vi "Connect.vi"(8 "error in (no error)":errorcluster, 11 "ImageHandler in":refnum<class "ImageHandler.lvclass">) -> (0 "error out":errorcluster, 1 "Serial Number":string, 2 "Sensor Status":i32, 3 "ImageHandler out":refnum<class "ImageHandler.lvclass">)   [LabVIEW 2022 SP3, in "ImageHandler.lvlib" / "ImageHandler.lvclass"]
uses:
  ImageHandler.lvclass
  C:/Program Files/National Instruments/LabVIEW 2022/vi.lib/ActorFramework/Actor/Actor.lvclass
  <vilib>/ActorFramework/Actor/Actor.lvclass/Actor.ctl
  ImageHandler.lvclass/ImageHandler.ctl
  ImageHandler - Controller -- Interface/ImageHandler - Controller -- Interface Messages/Log Message Msg/Log Message Msg.lvclass/Log Message Msg.ctl
  <vilib>/ActorFramework/Message Enqueuer/Message Enqueuer.lvclass/Message Enqueuer.ctl
  <vilib>/ActorFramework/Message Enqueuer/Enqueue.vi
  ImageHandler - Controller -- Interface/ImageHandler - Controller -- Interface Messages/Log Message Msg/Log Message Msg.lvclass
  C:/Program Files/National Instruments/LabVIEW 2022/vi.lib/ActorFramework/Message/Message.lvclass
  <vilib>/ActorFramework/Message Priority Queue/Priority Enqueue.vi
  BonTechDetector/BonTechDetector.lvlib
  <vilib>/ActorFramework/Actor/Actor.lvclass
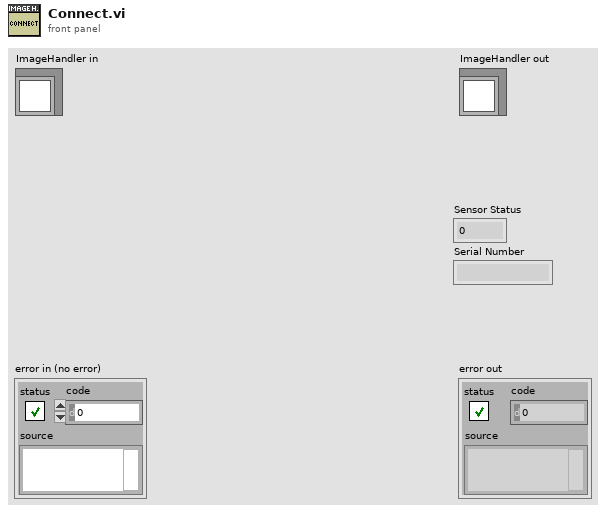
[diagram p1: front panel]
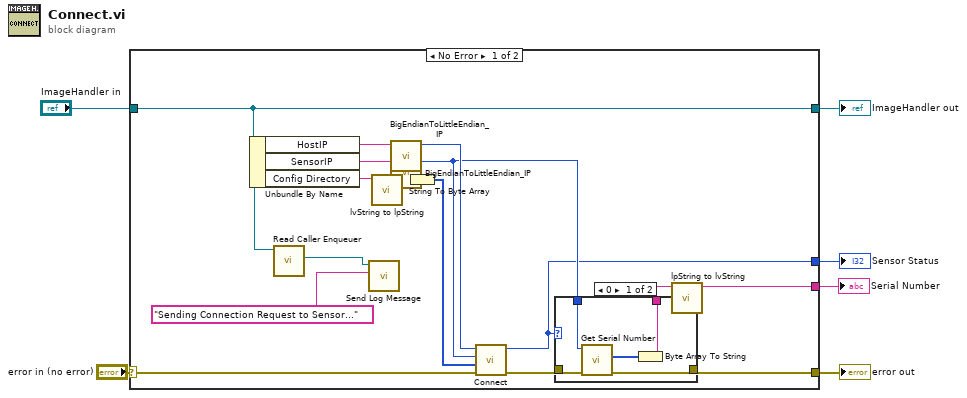
[diagram p0: block diagram]
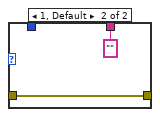
[diagram p2: hidden frame]
diagram:
  n1 = case shown="No Error" "error in (no error)" {
    selector: "error in (no error)" -> [w20 w31]
    tunnel: [w12 w31] -> w5
    tunnel: [w9 w30] -> w3
    tunnel: "ImageHandler in" -> [w9 w30]
    tunnel: [w10 _] -> w2
    tunnel: [w11 _] -> w1
    frame No Error {
      n2 = Unbundle By Name(w9) -> ("HostIP"=w22:string, "SensorIP"=w19:string, "Config Directory"=w18:string)
      n3 = call <vilib>:"Read Caller Enqueuer.vi"("Actor"=w9) -> ("Caller Enqueuer"=w8:refnum<class "Message Enqueuer.lvclass">)  [unwired: 10 in]
      n4 = call "Send Log Message.vi"("Log Message"="Sending Connection Request to Sensor...", "Message Enqueuer"=w8) -> ()  [unwired: 8 in, 2 out]
      n5 = call "lvString to lpString.vi"("LVString"=w18) -> ("LPTSTR String"=w17:string)  [unwired: 10 in]
      n6 = call "BigEndianToLittleEndian_IP.vi"("IP String"=w22) -> ("IP Network Order"=w21:u32)  [unwired: 10 in]
      n7 = call "BigEndianToLittleEndian_IP.vi"("IP String"=w19) -> ("IP Network Order"=w14:u32)  [unwired: 10 in]
      n8 = String To Byte Array(string=w17) -> (unsigned byte array=w16:u8[])
      n9 = call "Connect.vi"("error in (no error)"=w20, "ConfigDir"=w16, "nSensorIP"=w14, "nHostIP"=w21) -> ("error out"=w13:errorcluster, "function return"=w10:i32)  [unwired: 6 in]
      n10 = case shown="0" w10 {
        tunnel: [w27 "" ("string")] -> w15
        tunnel: w14 -> [w25 _]
        tunnel: w13 -> [w24 w29]
        tunnel: [w23 w29] -> w12
        frame 0 {
          n11 = call "Get Serial Number.vi"("error in (no error)"=w24, "nSensorIP"=w25) -> ("error out"=w23:errorcluster, "lpszSerialNum out"=w26:u8[])  [unwired: 7 in, 1 out]
          n12 = Byte Array To String(unsigned byte array=w26) -> (string=w27:string)
        }
        frame 1, Default {
        }
      }
      n13 = call "lpString to lvString.vi"("LPTSTR String"=w15) -> ("LVString"=w11:string)  [unwired: 10 in]
    }
    frame Error {
    }
  }
  "error out" <- w5
  "ImageHandler out" <- w3
  "Sensor Status" <- w2
  "Serial Number" <- w1
